vi "SpikeCounting_001.vi"(1 "Template":i32[](array[numeric]), 2 "Test object":i32[](array[numeric])) -> (0 "dissimiliarity":dbl)   [LabVIEW 2018]
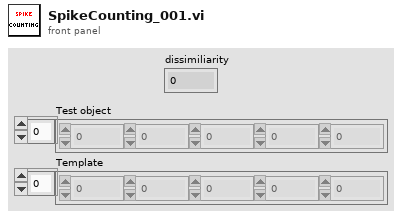
[diagram p1: front panel]
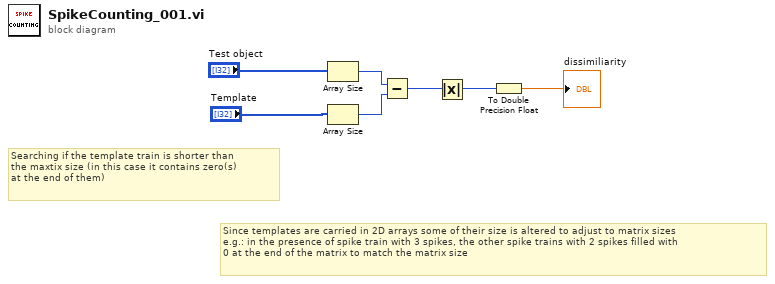
[diagram p0: block diagram]
diagram:
  # "Searching if the template train is shorter than \nthe maxtix size (in this case it contains zero(s)\nat the end of them)"
  # "Since templates are carried in 2D arrays some of their size is altered to adjust to matrix sizes\ne.g.: in the presence of spike train with 3 spikes, the other spike trains with 2 spikes filled with\n0 at the end of the matrix to match the matrix size"
  n1 = Array Size(array="Test object") -> (size(s)=w3:i32)
  n2 = Array Size(array="Template") -> (size(s)=w2:i32)
  n3 = Subtract(x=w3, y=w2) -> (x-y=w7:i32)
  n4 = Absolute Value(x=w7) -> (abs(x)=w4:i32)
  n5 = To Double Precision Float(number=w4) -> (double precision float=→"dissimiliarity":dbl)
